vi "UIEnableyesno.vi"(0 "CmdLib In":refnum<k24>, 5 "Status:":refnum<vi>, 9 "Device Array":T2(array[cluster]), 11 "error in":errorcluster) -> (15 "error out":errorcluster)   [LabVIEW 2021]
uses:
  Global Variablesyes.vi
  C:/Program Files/New Focus/New Focus Picomotor Application/Samples/LabVIEW/Model 8742/LabVIEW 2009/CmdLib.dll
  Program Files/New Focus/New Focus Picomotor Application/Samples/LabVIEW/Model 8742/LabVIEW 2009/CmdLib.dll
panel:
  in  "UI":T1
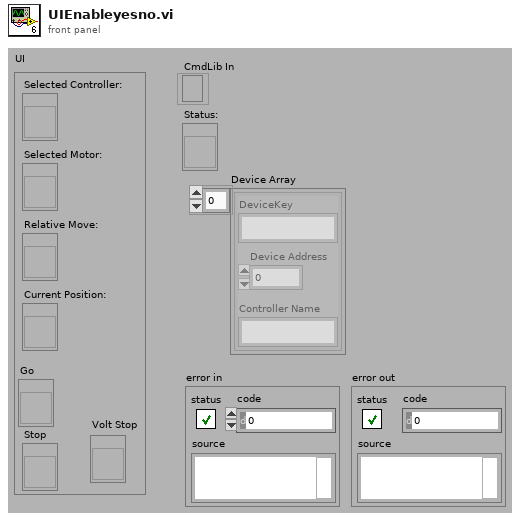
[diagram p1: front panel]
types:
  T1 = cluster{"Selected Controller:":refnum<vi>, "Selected Motor:":refnum<vi>, "Relative Move:":refnum<vi>, "Current Position:":refnum<vi>, "Go":refnum<vi>, "Stop":refnum<vi>, "Volt Stop":refnum<vi>}
  T2 = cluster{"DeviceKey":string, "Device Address":i32, "Controller Name":string}[]
  T3 = enum8{"Enabled", "Disabled", "Disabled and Grayed Out"}
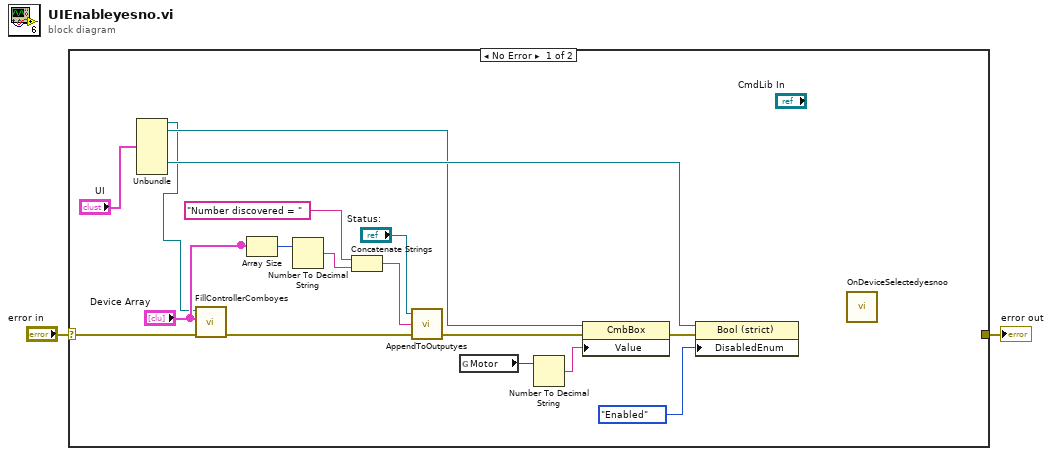
[diagram p0: block diagram]
diagram:
  n1 = case shown="No Error" "error in" {
    selector: "error in" -> [w15 w22]
    tunnel: [w17 w22] -> w2
    frame No Error {
      n2 = Unbundle("UI") -> ("Selected Controller:"=w4:refnum<vi>, "Selected Motor:"=w5:refnum<vi>, "Stop"=w6:refnum<vi>)  [unwired: 4 out]
      n3 = call "FillControllerComboyes.vi"("error in (no error)"=w15, "Device Array"="Device Array", "Selected Controller:"=w4) -> ("error out"=w14:errorcluster)  [unwired: 8 in]
      n4 = Array Size(array="Device Array") -> (size(s)=w16:i32)
      n5 = Number To Decimal String(number=w16) -> (decimal integer string=w19:string)  [unwired: 1 in]
      n6 = Concatenate Strings("Number discovered = " ("string"), w19) -> (w21:string)
      n7 = call "AppendToOutputyes.vi"("error in"=w14, "Input String"=w21, "Output Refnum In"="Status:") -> ("error out"=w9:errorcluster)  [unwired: 1 in, 1 out]
      n8 = global read "Global Variablesyes.vi" "Motor"() -> (w12:i32)
      n9 = Number To Decimal String(number=w12) -> (decimal integer string=w13:string)  [unwired: 1 in]
      n10 = property class="CmbBox"(reference=w5, error in=w9, "Value"=w13) -> (error out=w7:errorcluster)  [unwired: 1 out]
      n11 = property class="Bool (strict)"(reference=w6, error in=w7, "DisabledEnum"=T3."Enabled" ("Disabled")) -> ()  [unwired: 2 out]
      n12 = call "OnDeviceSelectedyesnoo.vi"() -> ()  [unwired: 11 in, 1 out]
    }
    frame Error {
    }
  }
  "error out" <- w2
